vi "Pre-Actor.vi"(8 "error in (no error)":errorcluster, 11 "FunctionGenerator in":refnum<class "FunctionGenerator.lvclass">) -> (0 "error out":errorcluster, 3 "FunctionGenerator out":refnum<class "FunctionGenerator.lvclass">)   [LabVIEW 2019, in "FunctionGenerator.lvlib" / "FunctionGenerator.lvclass"]
doc: "This override VI is to provide the means for children classes to perform application specific post launch initialization functions that must be performed *prior* to calling the actor. \n\n***DO NOT USE THE CHECK FOR FAULT ROUTINE HERE***"
uses:
  Library/FunctionGenerator.lvclass
  Library/FunctionGenerator.lvclass/FunctionGenerator.ctl
  builds/Instruments/Instruments.lvlibp/Library/Instruments.lvclass
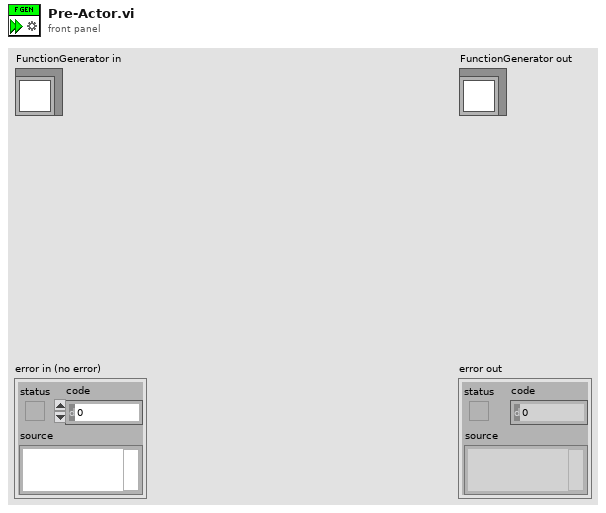
[diagram p1: front panel]
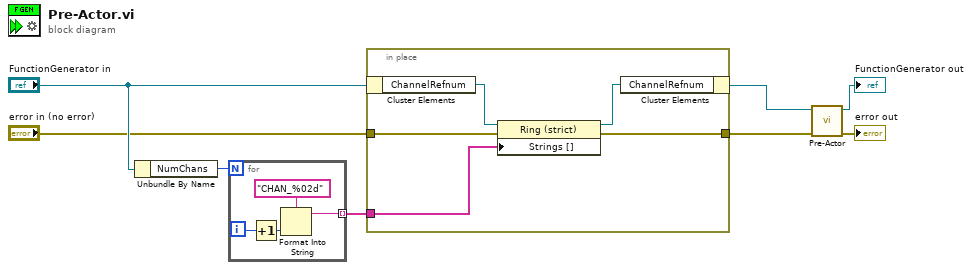
[diagram p0: block diagram]
diagram:
  n1 = Unbundle By Name("FunctionGenerator in") -> ("NumChans"=w6:i32)
  n2 = for {
    N: w6 -> [_]
    tunnel: [w9] -> w3 mode=indexing
    i -> [w11]
    n3 = Increment(x=w11) -> (x+1=w10:i32)
    n4 = Format Into String(format string="CHAN_%02d", w10) -> (resulting string=w9:string)  [unwired: 2 in, 1 out]
  }
  n5 = in-place {
    in-place-border: w3 -> [w15]
    in-place-border: "error in (no error)" -> [w14]
    in-place-border: [w13] -> w1
    n6 = in-place-cluster #1("FunctionGenerator in") -> ("ChannelRefnum"=w17:refnum<vi>)
    n7 = property class="Ring (strict)"(reference=w17, error in=w14, "Strings []"=w15) -> (reference out=w16:refnum<vi>, error out=w13:errorcluster)
    n8 = in-place-cluster #1("ChannelRefnum"=w16) -> (w4:refnum<class "FunctionGenerator.lvclass">)
  }
  n9 = call-parent "Pre-Actor.vi"("error in (no error)"=w1, "Instruments in"=w4) -> ("error out"=→"error out":errorcluster, "Instruments out"=→"FunctionGenerator out":refnum<class "FunctionGenerator.lvclass">)  [unwired: 8 in]
